vi "Enqueue.vi"(7 "Instance":i32, 8 "error in (no error)":errorcluster, 10 "Data":variant, 11 "Msg":string) -> (0 "error out":errorcluster)   [LabVIEW 2017, in "Communication.lvlib"]
uses:
  Communication.lvlib
  SubVIs/MsgData.ctl
  SubVIs/MsgAck.ctl
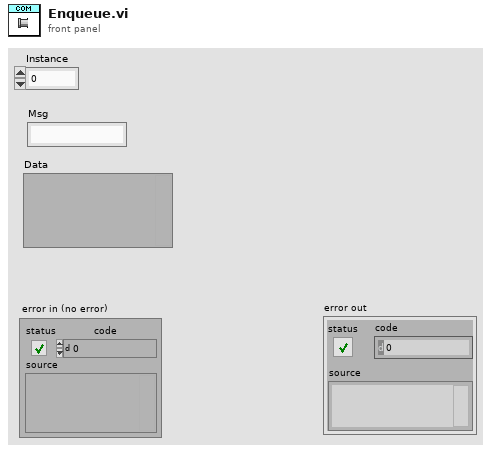
[diagram p1: front panel]
types:
  T1 = typedef "Communication.lvlib/MsgData.ctl" = cluster{"Msg":string, "Data":variant, "Ack":refnum<notifier>}
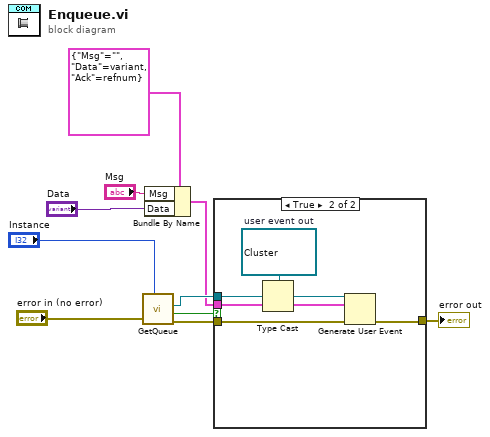
[diagram p0: block diagram]
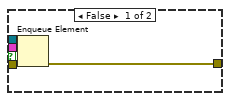
[diagram p2: hidden frame]
diagram:
  n1 = call "GetQueue.vi"("Instance"="Instance", "error in (no error)"="error in (no error)") -> ("error out"=w8:errorcluster, "Event?"=w1:bool, "queue out"=w7:refnum<queue>)  [unwired: 7 in]
  n2 = Bundle By Name(cluster=T1 {"Msg"="", "Data"=variant, "Ack"=refnum} ("element"), "Msg"="Msg", "Data"="Data") -> (w5:T1)
  n3 = case shown="True" w1 {
    tunnel: w8 -> [w14 w18]
    tunnel: w7 -> [w13 w20]
    tunnel: w5 -> [w12 w16]
    tunnel: [w11 w15] -> w2
    frame False {
      n4 = Enqueue Element(queue=w13, element=w12, error in (no error)=w14) -> (error out=w11:errorcluster)  [unwired: 1 in, 2 out]
    }
    frame True {
      w19 = refnum<user-event> refnum  # user event out
      n5 = Type Cast(type=w19, x=w20) -> (*(type *) &x=w17:refnum<user-event>)
      n6 = Generate User Event(user event=w17, event data cluster=w16, error in=w18) -> (error out=w15:errorcluster)  [unwired: 1 in, 1 out]
    }
  }
  "error out" <- w2
